vi "CaracterTecla_a_FrecuenciasDTMF.vi"(3 "Caracter_Tecla":string) -> (0 "Min_Frecuencia":dbl, 1 "Max_Frecuencia":dbl)   [LabVIEW 2018]
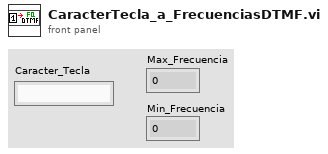
[diagram p1: front panel]
types:
  T1 = cluster{"Frecuencia_Alta":dbl, "Frecuencia_Baja":dbl, "Indicador_Tecla":dbl, "Tecla":string}[]
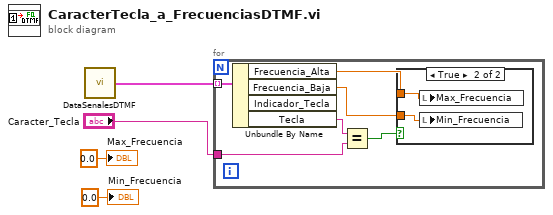
[diagram p0: block diagram]
diagram:
  n1 = call "DataSenalesDTMF.vi"() -> ("Data_Senales_DTMF"=w4:T1)  [unwired: 1 in]
  n2 = for {
    tunnel: w4 -> [w10] mode=indexing
    tunnel: "Caracter_Tecla" -> [w9]
    n3 = Unbundle By Name(w10) -> ("Frecuencia_Alta"=w6:dbl, "Frecuencia_Baja"=w5:dbl, "Tecla"=w8:string)  [unwired: 1 out]
    n4 = Equal?(x=w8, y=w9) -> (x = y?=w7:bool)
    n5 = case shown="True" w7 {
      tunnel: w6 -> [_ w12]
      tunnel: w5 -> [_ w11]
      frame False {
      }
      frame True {
        n6 = local write "Max_Frecuencia"(w12) -> ()
        n7 = local write "Min_Frecuencia"(w11) -> ()
      }
    }
  }
  "Max_Frecuencia" <- 0.0 ("Max_Frecuencia")
  "Min_Frecuencia" <- 0.0 ("Min_Frecuencia")
